vi "Translator.TranslateThis.vi"(7 "Language (English)":string="English", 8 "error in":errorcluster, 11 "vi reference":refnum<vi>) -> (0 "error out":errorcluster)   [LabVIEW 2016]
uses:
  Global/ApplicationGlobal.vi
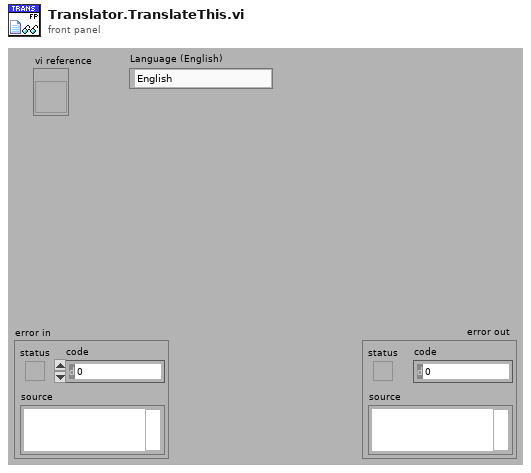
[diagram p1: front panel]
types:
  T1 = typedef "Translator.ControlData.ctl" = cluster{"ref":refnum<vi>, "strict?":bool, "save font?":bool, "type":T2, "root":string, "label":string, "caption":string, "bln.false":string, "bln.true":string, "cols":string[], "rows":string[]}
  T2 = typedef "Translator.ControlTypes.ctl" = enum16{"Cluster", "Array", "Boolean", "Ring", "String", "Tab", "Listbox", "Multicolumn listbox", "Table", "Tree", "Other"}
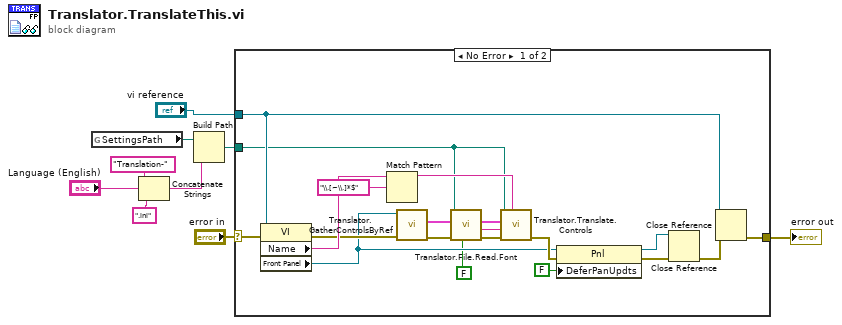
[diagram p0: block diagram]
diagram:
  n1 = global read "ApplicationGlobal.vi" "SettingsPath"() -> (w4:path)
  n2 = Concatenate Strings("Translation-" ("string"), "Language (English)", ".ini" ("string")) -> (w5:string)
  n3 = Build Path(base path=w4, name or relative path=w5) -> (appended path=w3:path)
  n4 = case shown="No Error" "error in" {
    selector: "error in" -> [w26 w29]
    tunnel: w3 -> [w15 _]
    tunnel: "vi reference" -> [w17 _]
    tunnel: [w21 w29] -> w8
    frame No Error {
      n5 = property class="VI"(reference=w17, error in=w26) -> (error out=w12:errorcluster, "Name"=w20:string, "Front Panel"=w11:refnum<vi>)  [unwired: 1 out]
      n6 = Match Pattern(string=w20, regular expression="\\.[~\\.]*$") -> (before substring=w19:string)  [unwired: 4 out]
      n7 = call "Translator.GatherControlsByRef.vi"("error in"=w12, "Front Panel"=w11) -> ("error out"=w14:errorcluster, "Controls out"=w27:T1[])  [unwired: 8 in]
      n8 = call "Translator.File.Read.Font.vi"("Do not save font? (F)"=FALSE, "error in"=w14, "Translation file"=w15) -> ("error out"=w13:errorcluster, "font name"=w16:string)  [unwired: 6 in, 1 out]
      n9 = call "Translator.Translate.Controls.vi"("group"=w19, "error in"=w13, "font name"=w16, "Controls out"=w27, "Translation file"=w15) -> ("error out"=w18:errorcluster)  [unwired: 6 in]
      n10 = property class="Pnl"(reference=w11, error in=w18, "DeferPanUpdts"=FALSE ("Defer Panel Updates")) -> (reference out=w25:refnum<vi>, error out=w24:errorcluster)
      n11 = Close Reference(reference=w25, error in (no error)=w24) -> (error out=w22:errorcluster)
      n12 = Close Reference(reference=w17, error in (no error)=w22) -> (error out=w21:errorcluster)
    }
    frame Error {
    }
  }
  "error out" <- w8
